vi "Utility Multiple Write To Registers in Configuration Mode.vi"(0 "VISA resource name":refnum<visa-resource-name>, 1 "Unit Address (1)":u8=1, 5 "Registers Addresses (0)":u16[](array[numeric])=[0, 123, 124, 54, 128], 7 "Data (0)":i16[](array[numeric]), 11 "error in (no error)":errorcluster) -> (4 "VISA resource name out":refnum<visa-resource-name>, 15 "error out":errorcluster)   [LabVIEW 2010, in "Eurotherm 32xx Series.lvlib"]
doc: "This VI writes the values to the specified registers of specified unit in device configuration mode."
uses:
  <instrlib>/Eurotherm 32xx Series/Eurotherm 32xx Series.lvlib
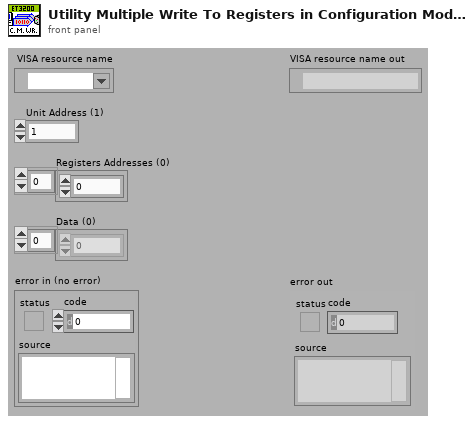
[diagram p1: front panel]
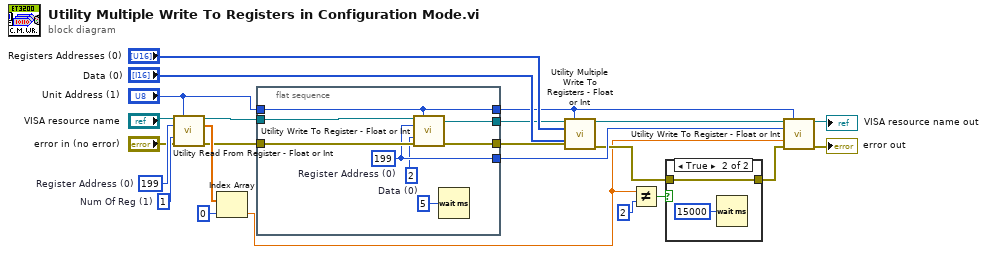
[diagram p0: block diagram]
diagram:
  w22 = u16 199  # Register Address (0)
  w23 = u16 1  # Num Of Reg (1)
  n1 = call <instrlib>:"Utility Read From Register - Float or Int.vi"("VISA resource name"="VISA resource name", "Unit Address (1)"="Unit Address (1)", "Register Address (0)"=w22, "Num Of Reg (1)"=w23, "error in (no error)"="error in (no error)") -> ("VISA resource name out"=w14:refnum<visa-resource-name>, "Data"=w21:sgl[], "error out"=w13:errorcluster)  [unwired: 8 in]
  n2 = Index Array(array=w21, index=0) -> (element=w3:sgl)
  n3 = flat-sequence {
    tunnel: [w24] -> w7
    tunnel: [w27] -> w10
    tunnel: [w28] -> w11
    tunnel: [w29] -> w12
    tunnel: w14 -> [w31]
    tunnel: w13 -> [w30]
    tunnel: "Unit Address (1)" -> [w24]
    frame #0 {
      w26 = i16 2  # Data (0)
      w27 = u16 199  # Register Address (0)
      n4 = call <instrlib>:"Utility Write To Register - Float or Int.vi"("VISA resource name"=w31, "Unit Address (1)"=w24, "Register Address (0)"=w27, "Data (0)"=w26, "error in (no error)"=w30) -> ("VISA resource name out"=w28:refnum<visa-resource-name>, "error out"=w29:errorcluster)  [unwired: 9 in]
      n5 = Wait (ms)(milliseconds to wait=u32 5) -> ()  [unwired: 1 out]
    }
  }
  n6 = call <instrlib>:"Utility Multiple Write To Registers - Float or Int.vi"("VISA resource name"=w11, "Unit Address (1)"=w7, "Registers Addresses (0)"="Registers Addresses (0)", "Data (0)"="Data (0)", "error in (no error)"=w12) -> ("VISA resource name out"=w15:refnum<visa-resource-name>, "error out"=w4:errorcluster)  [unwired: 9 in]
  n7 = Not Equal?(x=w3, y=i16 2) -> (x != y?=w1:bool)
  n8 = case shown="True" w1 {
    tunnel: [w32 w33] -> w5
    tunnel: w4 -> [w32 w33]
    frame False {
    }
    frame True {
      n9 = Wait (ms)(milliseconds to wait=u32 15000) -> ()  [unwired: 1 out]
    }
  }
  n10 = call <instrlib>:"Utility Write To Register - Float or Int.vi"("VISA resource name"=w15, "Unit Address (1)"=w7, "Register Address (0)"=w10, "Data (0)"=w3, "error in (no error)"=w5) -> ("VISA resource name out"=→"VISA resource name out":refnum<visa-resource-name>, "error out"=→"error out":errorcluster)  [unwired: 9 in]
